vi "feed_sound_output.vi"(5 "Output buffer feeds [1/sec]":u16, 6 "Ctl Refnum":refnum<vi>, 7 "Input buffer length [sec]":dbl, 8 "error in (no error)":errorcluster, 9 "sound format":T1={"sample rate (S/s)"=48000.0, "number of channels"=1, "bits per sample"=16}, 10 "Queue":refnum<queue>, 11 "task ID":T2 format="%.0x") -> (0 "error out":errorcluster)   [LabVIEW 2011]
uses:
  <vilib>/sound2/lvsound2.llb/Sound Output Task ID.ctl
  <vilib>/sound2/lvsound2.llb/Sound Data Format.ctl
  <vilib>/sound2/lvsound2.llb/Sound Output Write (DBL Single).vi
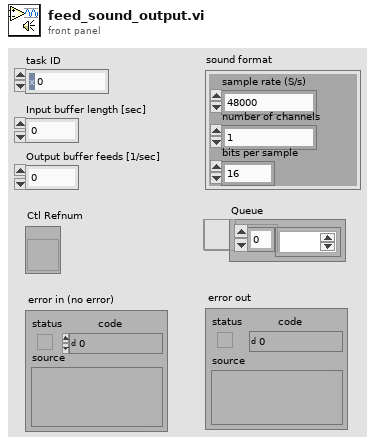
[diagram p1: front panel]
types:
  T1 = typedef "Sound Data Format.ctl" = cluster{"sample rate (S/s)":dbl, "number of channels":i32, "bits per sample":i32}
  T2 = typedef "Sound Output Task ID.ctl" = u32
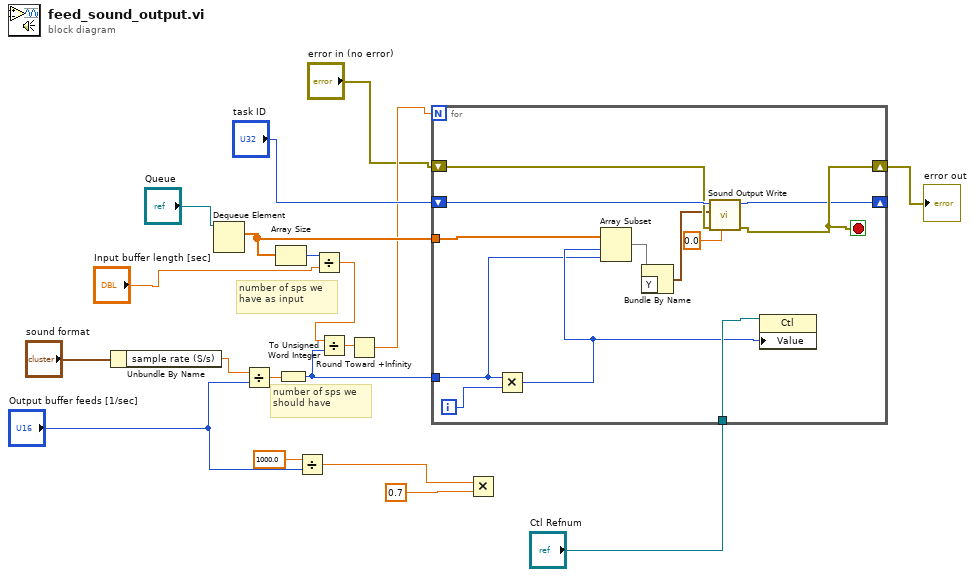
[diagram p0: block diagram]
diagram:
  # "number of sps we have as input"
  # "number of sps we should have"
  n1 = Unbundle By Name("sound format") -> ("sample rate (S/s)"=w13:dbl)
  n2 = Dequeue Element(queue="Queue") -> (element=w17:dbl[])  [unwired: 2 in, 3 out]
  n3 = Divide(x=w13, y="Output buffer feeds [1/sec]") -> (x/y=w9:dbl)
  n4 = Array Size(array=w17) -> (size(s)=w16:i32)
  n5 = To Unsigned Word Integer(number=w9) -> (unsigned 16bit integer=w8:u16)
  n6 = Divide(x=1000.0, y="Output buffer feeds [1/sec]") -> (x/y=w3:dbl)
  n7 = Divide(x=w16, y="Input buffer length [sec]") -> (x/y=w12:dbl)
  n8 = Divide(x=w12, y=w8) -> (x/y=w11:dbl)
  n9 = Round Toward +Infinity(x=w11) -> (ceil(x): smallest int >= x=w10:dbl)
  n10 = for {
    N: w10 -> [_]
    tunnel: w17 -> [w30]
    tunnel: w8 -> [w23]
    shift-right: [w27] -> w7
    shift-left: "error in (no error)" -> [w28]
    shift-right: [w26] -> _
    shift-left: "task ID" -> [w31]
    tunnel: "Ctl Refnum" -> [w25]
    i -> [w29]
    stop <- w27 stop-if-true
    n11 = Multiply(x=w23, y=w29) -> (x*y=w24:i32)
    n12 = Array Subset(array=w30, index=w24, length=w23) -> (w20:dbl[])
    n13 = Bundle By Name("Y"=w20) -> (w21:waveform(dbl))  [unwired: 1 in]
    n14 = call-poly <vilib>:"Sound Output Write.vi"("timeout (sec)"=0.0, "error in (no error)"=w28, "data"=w21, "task ID"=w31) -> ("error out"=w27:errorcluster, "task ID out"=w26:T2)  [unwired: 6 in]
    n15 = property on="Property Node" class="Ctl"(reference=w25, "Value"=w24) -> ()  [unwired: 1 in, 2 out]
  }
  "error out" <- w7
  n16 = Multiply(x=w3, y=0.7) -> ()  [unwired: 1 out]
